vi "Parity_Calc_Validator.vi"() -> ()   [LabVIEW 2012]
panel:
  out "Odd2?":bool
  out "Numeric 2":u32 format="%.0b"
  out "Odd?":bool
  in  "Numeric":u32
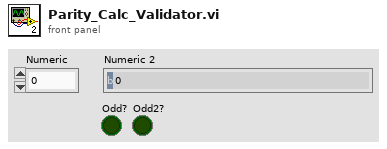
[diagram p1: front panel]
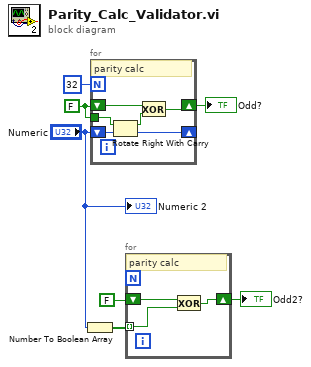
[diagram p0: block diagram]
diagram:
  w7 = FALSE
  n1 = Number To Boolean Array(number="Numeric") -> (Boolean array=w3:bool[])
  n2 = for {
    N: 32 -> [_]
    shift-right: [w13] -> w5
    shift-left: w7 -> [w12]
    shift-right: [w10] -> _
    shift-left: "Numeric" -> [w11]
    tunnel: w7 -> [w9]
    # "parity calc"
    n3 = Rotate Right With Carry(2:w11, 3:w9) -> (0:w10:u32, 1:w8:bool)
    n4 = Exclusive Or(1:w8, 2:w12) -> (0:w13:bool)
  }
  "Odd?" <- w5
  n5 = for {
    shift-right: [w16] -> w1
    shift-left: FALSE -> [w15]
    tunnel: w3 -> [w14] mode=indexing
    # "parity calc"
    n6 = Exclusive Or(1:w14, 2:w15) -> (0:w16:bool)
  }
  "Odd2?" <- w1
  "Numeric 2" <- "Numeric"
